vi "meta range clip.vi"(7 "result_out":dbl, 8 "error in (no error)":errorcluster, 9 "clip_step":i32, 10 "value":dbl, 11 "h":u64) -> (0 "error out":errorcluster, 3 "function return":u32(ring), 5 "result_out out":dbl)   [LabVIEW 2023, in "uhd.lvlib"]
doc: "UHD_API uhd_error uhd_meta_range_clip(\n uhd_meta_range_handle h, double value, bool clip_step, double* result_out);"
uses:
  <userlib>/uhd/uhd.lvlib
  <userlib>/uhd/uhd.dll
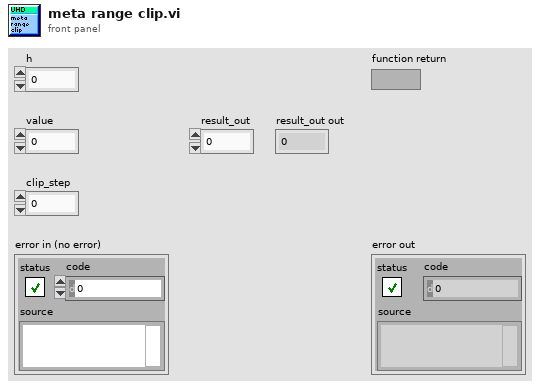
[diagram p1: front panel]
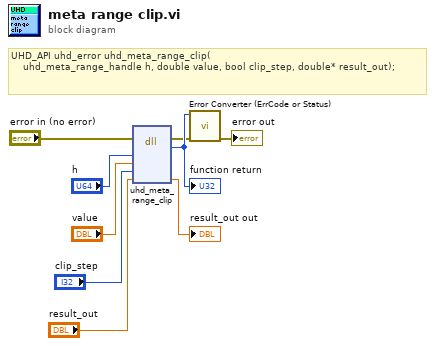
[diagram p0: block diagram]
diagram:
  # "UHD_API uhd_error uhd_meta_range_clip(\n    uhd_meta_range_handle h, double value, bool clip_step, double* result_out);"
  n1 = dll-call lib="C:/Program Files/National Instruments/LabVIEW 2023/user.lib/uhd/uhd.*" fn="uhd_meta_range_clip"(error in="error in (no error)", "h"="h", "value"="value", "clip_step"="clip_step", "result_out"="result_out") -> (error out=w2:errorcluster, w9:u32, "result_out"=→"result_out out":dbl)  [unwired: 5 in, 1 out]
  "function return" <- w9
  n2 = call <userlib>:"Error Converter (ErrCode or Status).vi"("error in (no error)"=w2, "error code"=w9) -> ("error out"=→"error out":errorcluster)  [unwired: 9 in]
